vi "String - Remove Front 0xFFFEs(2).vi"(11 "Sting IN":string="ÿþ«Í\u00124ÿþVxÜþ") -> (3 "String OUT":string)   [LabVIEW 2013]
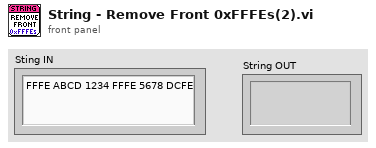
[diagram p1: front panel]
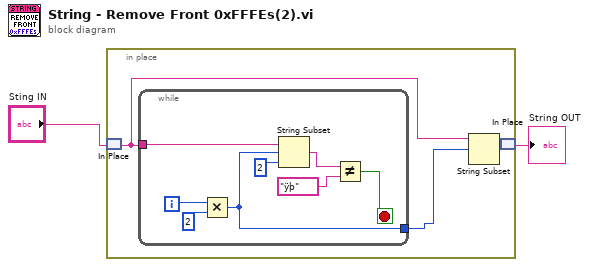
[diagram p0: block diagram]
diagram:
  n1 = in-place {
    n2 = in-place-match #1("Sting IN") -> (w4:string)
    n3 = while {
      tunnel: w4 -> [w13]
      tunnel: [w6] -> w3
      i -> [w9]
      stop <- w7 stop-if-true
      n4 = Multiply(x=w9, y=2) -> (x*y=w6:i32)
      n5 = String Subset(string=w13, offset (0)=w6, length (rest)=2 ("length (rest)")) -> (substring=w10:string)
      n6 = Not Equal?(x=w10, y="ÿþ" ("string")) -> (x != y?=w7:bool)
    }
    n7 = String Subset(string=w4, offset (0)=w3) -> (substring=w5:string)  [unwired: 1 in]
    n8 = in-place-match #1(w5) -> (→"String OUT":string)
  }
